vi "GenerateTriggeredStimulus.vi"(8 "error in (no error)":errorcluster, 11 "Stimulus in":refnum<class "HeadorTailRails.lvclass">) -> (0 "error out":errorcluster, 2 "TriggeredStimulus":sgl[][](array[numeric]), 3 "Stimulus out":refnum<class "HeadorTailRails.lvclass">)   [LabVIEW 2019, in "HeadorTailRails.lvclass"]
uses:
  HeadorTailRails.lvclass
  HeadorTailRails.lvclass/HeadorTailRails.ctl
  ParametersGlobal.vi
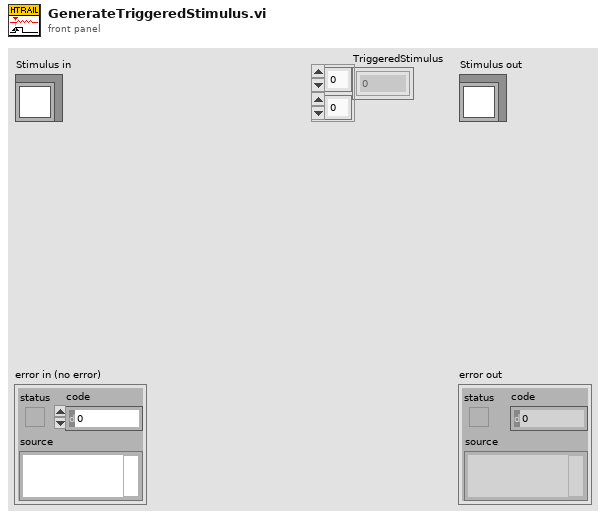
[diagram p1: front panel]
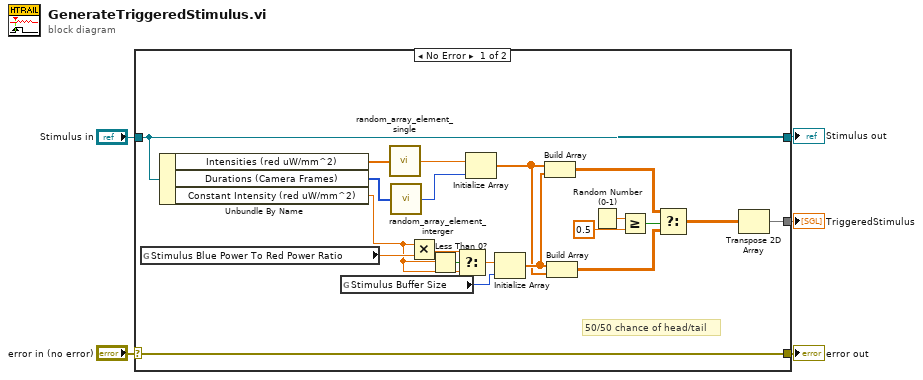
[diagram p0: block diagram]
diagram:
  n1 = case shown="No Error" "error in (no error)" {
    selector: "error in (no error)" -> [w26 w28]
    tunnel: [w26 w28] -> w3
    tunnel: [w15 w27] -> w1
    tunnel: "Stimulus in" -> [w15 w27]
    tunnel: [w21 _] -> w2
    frame No Error {
      # "50/50 chance of head/tail"
      n2 = global read "ParametersGlobal.vi" "Stimulus Blue Power To Red Power Ratio"() -> (w18:sgl)
      n3 = Unbundle By Name(w15) -> ("Intensities (red uW/mm^2)"=w25:sgl[], "Durations (Camera Frames)"=w24:i32[], "Constant Intensity (red uW/mm^2)"=w14:sgl)
      n4 = global read "ParametersGlobal.vi" "Stimulus Buffer Size"() -> (w16:i32)
      n5 = call "random_array_element_single.vi"("Array of numbers"=w25) -> ("Randomly selected number"=w23:sgl)
      n6 = call "random_array_element_interger.vi"("Array of numbers"=w24) -> ("Randomly selected number"=w22:i32)
      n7 = Multiply(x=w14, y=w18) -> (x*y=w20:sgl)
      n8 = Less Than 0?(x=w14) -> (x < 0?=w19:bool)
      n9 = Select(t=w20, s=w19, f=w14) -> (s? t:f=w17:sgl)
      n10 = Initialize Array(w23, w22) -> (w9:sgl[])
      n11 = Initialize Array(w17, w16) -> (w10:sgl[])
      n12 = Build Array(w9, w10) -> (w8:sgl[][])
      n13 = Build Array(w10, w9) -> (w7:sgl[][])
      n14 = Random Number (0-1)() -> (number: 0 to 1=w13:dbl)
      n15 = Greater Or Equal?(x=w13, y=0.5) -> (x >= y?=w11:bool)
      n16 = Select(t=w8, s=w11, f=w7) -> (s? t:f=w6:sgl[][])
      n17 = Transpose 2D Array(2D array=w6) -> (transposed array=w21:sgl[][])
    }
    frame Error {
    }
  }
  "error out" <- w3
  "Stimulus out" <- w1
  "TriggeredStimulus" <- w2
